vi "Set Setpoint.vi"(8 "error in (no error)":errorcluster, 9 "Setpoint (%)":dbl, 11 "Bronkhorst Settings in":T1={"VISA resource name"="", "Simulated?"=FALSE, "Smoothing Steps"=1} {"Smoothing Steps" min=1 step=1}) -> (0 "error out":errorcluster, 1 "Connection Error":bool, 3 "Bronkhorst Settings out":T1={"VISA resource name"="", "Simulated?"=FALSE, "Smoothing Steps"=1} {"Smoothing Steps" min=1 step=1})   [LabVIEW 2021]
uses:
  Bronkhorst M13 Flow Meter/Settings Cluster.ctl
  <vilib>/regexp/Match Regular Expression.xnode
  Bronkhorst M13 Flow Meter/Bronkhorst M13 Flow Meter.lvlib
panel:
  out "whole match":string
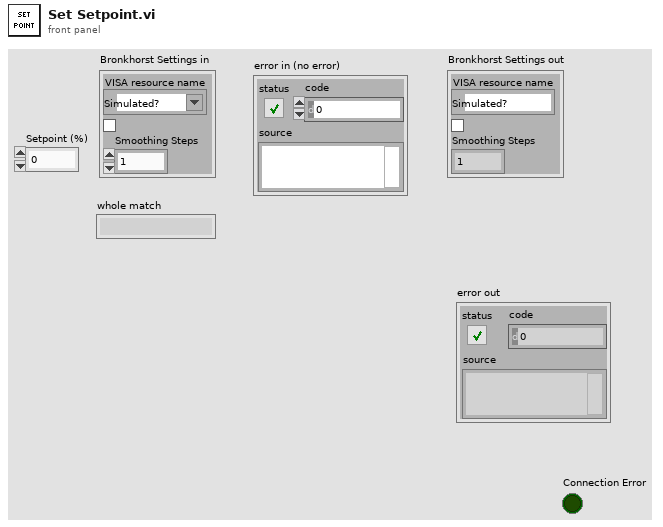
[diagram p1: front panel]
types:
  T1 = typedef "Bronkhorst M13 Flow Meter.lvlib/Settings Cluster.ctl" = cluster{"VISA resource name":refnum<visa-resource-name>, "Simulated?":bool, "Smoothing Steps":i32}
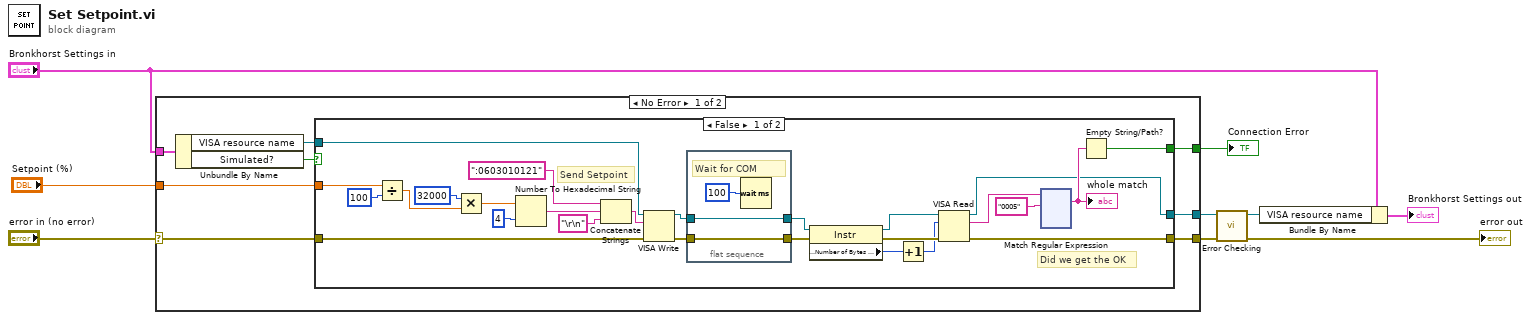
[diagram p0: block diagram]
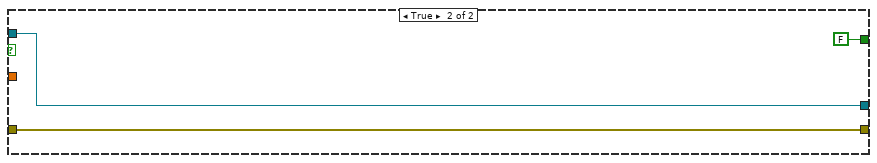
[diagram p2: hidden frame]
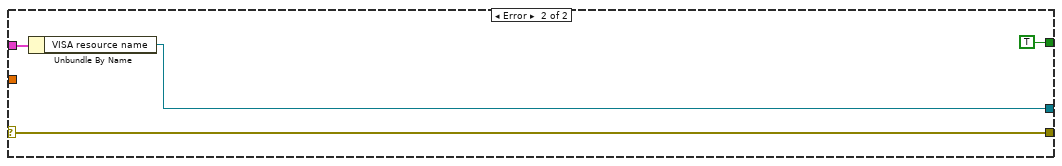
[diagram p3: hidden frame]
diagram:
  n1 = case shown="No Error" "error in (no error)" {
    selector: "error in (no error)" -> [w16 w170]
    tunnel: [w15 w170] -> w4
    tunnel: "Bronkhorst Settings in" -> [w14 w169]
    tunnel: [w12 w168] -> w6
    tunnel: "Setpoint (%)" -> [w11 _]
    tunnel: [w10 TRUE] -> w1
    frame No Error {
      n2 = Unbundle By Name(w14) -> ("VISA resource name"=w13:refnum<visa-resource-name>, "Simulated?"=w17:bool)
      n3 = case shown="False" w17 {
        tunnel: [w31 w166] -> w15
        tunnel: w16 -> [w35 w166]
        tunnel: [w24 w165] -> w12
        tunnel: w13 -> [w36 w165]
        tunnel: w11 -> [w21 _]
        tunnel: [w23 FALSE] -> w10
        frame False {
          # "Did we get the OK"
          # "Send Setpoint"
          n4 = Divide(x=w21, y=100) -> (x/y=w20:dbl)
          n5 = Multiply(x=32000, y=w20) -> (x*y=w18:dbl)
          n6 = Number To Hexadecimal String(1:i16 4 ("width (-)"), 2:w18) -> (0:w27:string)
          n7 = Concatenate Strings(":0603010121" ("Command"), w27, "\r\n") -> (w28:string)
          n8 = VISA Write(VISA resource name=w36, write buffer=w28, error in (no error)=w35) -> (VISA resource name out=w41:refnum<visa-resource-name>, error out=w39:errorcluster)  [unwired: 1 out]
          n9 = flat-sequence {
            tunnel: [w163] -> w40
            tunnel: w41 -> [w163]
            tunnel: [w162] -> w38
            tunnel: w39 -> [w162]
            frame #0 {
              # "Wait for COM"
              n10 = Wait (ms)(milliseconds to wait=u32 100) -> ()  [unwired: 1 out]
            }
          }
          n11 = property class="Instr"(reference=w40, error in=w38) -> (reference out=w43:refnum<visa-resource-name>, error out=w42:errorcluster, "Serial Settings:Number of Bytes at Serial Port"=w33:u32)
          n12 = Increment(x=w33) -> (x+1=w32:u32)
          n13 = VISA Read(VISA resource name=w43, byte count=w32, error in (no error)=w42) -> (VISA resource name out=w24:refnum<visa-resource-name>, read buffer=w34:string, error out=w31:errorcluster)  [unwired: 1 out]
          n14 = xnode "Match Regular Expression"("input string"=w34, "regular expression"="0005" ("Regular Expression for Extracting Weight")) -> ("whole match"=w25:string)  [unwired: 4 in, 4 out]
          "whole match" <- w25
          n15 = Empty String/Path?(string/path=w25) -> (empty?=w23:bool)
        }
        frame True {
        }
      }
    }
    frame Error {
      n16 = Unbundle By Name(w169) -> ("VISA resource name"=w168:refnum<visa-resource-name>)
    }
  }
  "Connection Error" <- w1
  n17 = call "Error Checking.vi"("error in (no error)"=w4, "VISA resource name"=w6) -> ("error out"=→"error out":errorcluster, "VISA resource name"=w5:refnum<visa-resource-name>)  [unwired: 7 in, 1 out]
  n18 = Bundle By Name(cluster="Bronkhorst Settings in", "VISA resource name"=w5) -> (→"Bronkhorst Settings out":T1)
